vi "Read Event Ref.vi"(8 "error in":errorcluster, 11 "simple_html_chat_ui in":refnum<class "simple_html_chat_ui.lvclass">) -> (0 "error out":errorcluster, 2 "Event Ref":refnum<user-event>, 3 "simple_html_chat_ui out":refnum<class "simple_html_chat_ui.lvclass">)   [LabVIEW 2020, in "simple_html_chat_ui.lvclass"]
uses:
  simple_html_chat_ui.lvclass
  typedefs/event_data.ctl
  simple_html_chat_ui.lvclass/simple_html_chat_ui.ctl
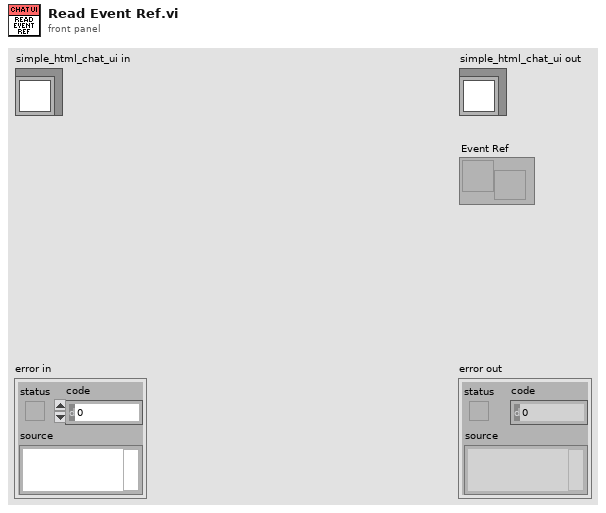
[diagram p1: front panel]
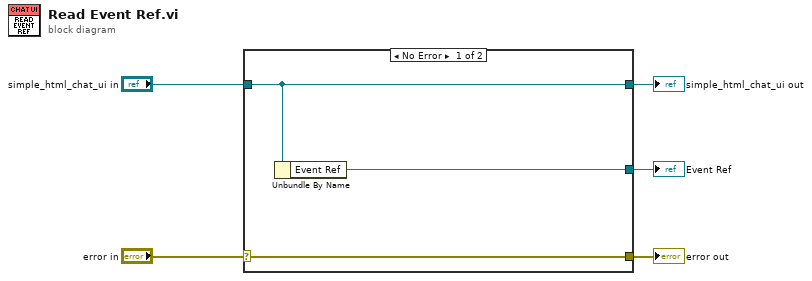
[diagram p0: block diagram]
diagram:
  n1 = case shown="No Error" "error in" {
    selector: "error in" -> [w8 w9]
    tunnel: [w8 w9] -> w4
    tunnel: [w7 w10] -> w2
    tunnel: "simple_html_chat_ui in" -> [w7 w10]
    tunnel: [w6 _] -> w1
    frame No Error {
      n2 = Unbundle By Name(w7) -> ("Event Ref"=w6:refnum<user-event>)
    }
    frame Error {
    }
  }
  "error out" <- w4
  "simple_html_chat_ui out" <- w2
  "Event Ref" <- w1
